vi "保存数据.vi"   [LabVIEW 2016, in "main.lvlib"]
uses:
  main.lvlib
types:
  T1 = typedef "剖面数据_EXO2.ctl" = cluster{"时间":timestamp, "测量模式":string, "数据类型":string, "数据标识":string, "湖面水深":sgl, "缆绳下放长度":sgl, "层数":u16, "row":u16, "水温":sgl, "比电导率":sgl, "电导率":sgl, "盐度":sgl, "总溶解固体":sgl, "pH":sgl, "pHmV":sgl, "ORP":sgl, "饱和度":sgl, "DO":sgl, "浊度":sgl, "叶绿素a":sgl, "蓝绿藻":sgl, "水深":sgl, "设置水深":sgl}
  T2 = typedef "剖面数据_bbe_NAQDO.ctl" = cluster{"时间":timestamp, "测量模式":string, "数据类型":string, "数据标识":string, "湖面水深":sgl, "缆绳下放长度":sgl, "层数":u16, "row":u16, "水温":sgl, "DO":sgl, "饱和度":sgl, "绿藻":sgl, "蓝藻":sgl, "硅甲藻":sgl, "隐藻":sgl, "黄色物质":sgl, "总藻":sgl, "透光率":sgl, "水深":sgl, "设置水深":sgl}
  T3 = cluster{"EXO2 message":T1, "bbe message":T2, "初级生产力":cluster{"时间":timestamp, "设置水深":sgl, "测控模式":u16, "系统状态":u16, "命令集":u16, "测量更新标志":u16, "测量平均次数":u16, "脉冲间歇时间":u16, "PMT增益":u16, "激发诱导光强":u16, "仿真环境光强":u16, "驰豫脉冲脉宽":u16, "驰豫脉冲周期":u16, "暗适应时间":u16, "光适应时间":u16, "系统电压":sgl, "系统温度":sgl, "F0":sgl, "Fm":sgl, "Fv/Fm":sgl, "σPSII":sgl, "τQA":sgl, "F0'":sgl, "Fm'":sgl, "Fv'":sgl, "Fv'/Fm'":sgl, "σPSII’":sgl, "τQA’":sgl, "Chla":sgl, "PAR":sgl, "GPP":sgl, "DF0":sgl, "DFv":sgl}}
  T4 = cluster{"时间":timestamp, "设置水深":sgl, "测控模式":u16, "系统状态":u16, "命令集":u16, "测量更新标志":u16, "测量平均次数":u16, "脉冲间歇时间":u16, "PMT增益":u16, "激发诱导光强":u16, "仿真环境光强":u16, "驰豫脉冲脉宽":u16, "驰豫脉冲周期":u16, "暗适应时间":u16, "光适应时间":u16, "系统电压":sgl, "系统温度":sgl, "F0":sgl, "Fm":sgl, "Fv/Fm":sgl, "σPSII":sgl, "τQA":sgl, "F0'":sgl, "Fm'":sgl, "Fv'":sgl, "Fv'/Fm'":sgl, "σPSII’":sgl, "τQA’":sgl, "Chla":sgl, "PAR":sgl, "GPP":sgl, "DF0":sgl, "DFv":sgl}
  T5 = typedef "checkbox.ctl" = bool
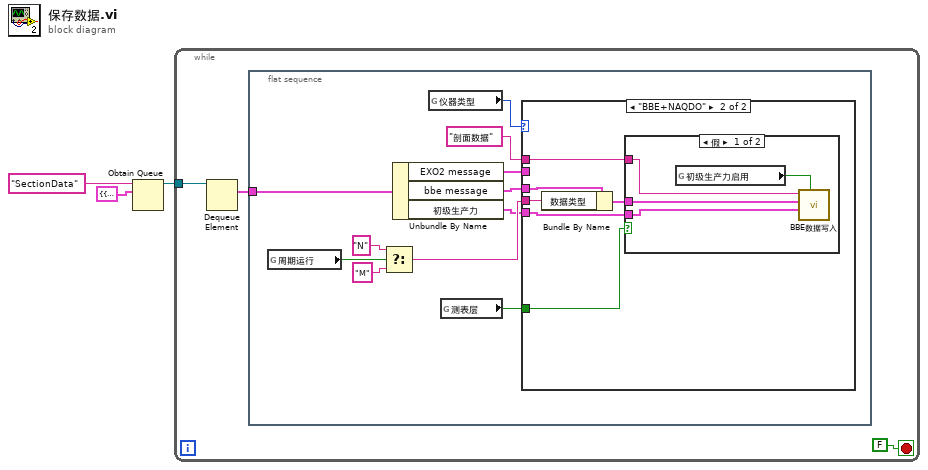
[diagram p0: block diagram]
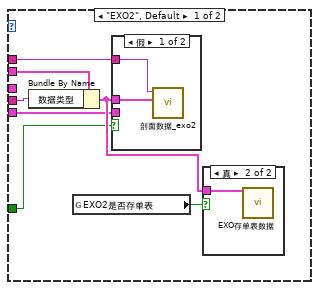
[diagram p2: hidden frame]
diagram:
  n1 = Obtain Queue(name (unnamed)="SectionData" ("名称（未命名）"), element data type=T3 {"EXO2 message"={"时间"=timestamp(0 s since 1904-01-01), "测量模式"="水样测试", "数据类型"="N", "数据标识"="N", "湖面水深"=0.0, "缆绳下放长度"=0.0, "层数"=0, "row"=0, "水温"=0.0, "比电导率"=0.0, "电导率"=0.0, "盐度"=0.0, "总溶解固体"=0.0, "pH"=0.0, "pHmV"=0.0, "ORP"=0.0, "饱和度"=0.0, "DO"=0.0, "浊度"=0.0, "叶绿素a"=0.0, "蓝绿藻"=0.0, "水深"=0.0, "设置水深"=0.0}, "bbe message"={"时间"=timestamp(0 s since 1904-01-01), "测量模式"="水样测试", "数据类型"="N", "数据标识"="N", "湖面水深"=0.0, "缆绳下放长度"=0.0, "层数"=0, "row"=0, "水温"=0.0, "DO"=0.0, "饱和度"=0.0, "绿藻"=0.0, "蓝藻"=0.0, "硅甲藻"=0.0, "隐藻"=0.0, "黄色物质"=0.0, "总藻"=0.0, "透光率"=0.0, "水深"=0.0, "设置水深"=0.0}, "初级生产力"={"时间"=timestamp(0 s since 1904-01-01), "设置水深"=0.0, "测控模式"=0, "系统状态"=0, "命令集"=0, "测量更新标志"=0, "测量平均次数"=0, "脉冲间歇时间"=0, "PMT增益"=0, "激发诱导光强"=0, "仿真环境光强"=0, "驰豫脉冲脉宽"=0, "驰豫脉冲周期"=0, "暗适应时间"=0, "光适应时间"=0, "系统电压"=0.0, "系统温度"=0.0, "F0"=0.0, "Fm"=0.0, "Fv/Fm"=0.0, "σPSII"=0.0, "τQA"=0.0, "F0'"=0.0, "Fm'"=0.0, "Fv'"=0.0, "Fv'/Fm'"=0.0, "σPSII’"=0.0, "τQA’"=0.0, "Chla"=0.0, "PAR"=0.0, "GPP"=0.0, "DF0"=0.0, "DFv"=0.0}} ("簇")) -> (queue out=w2:refnum<queue>)  [unwired: 3 in, 2 out]
  n2 = while {
    tunnel: w2 -> [w6]
    stop <- FALSE stop-if-true
    n3 = Dequeue Element(queue=w6) -> (element=w4:T3)  [unwired: 2 in, 3 out]
    n4 = flat-sequence {
      tunnel: w4 -> [w17]
      frame #0 {
        n5 = global read "全局断电保存变量.vi" "周期运行"() -> (w13:bool)
        n6 = Select(t="N" ("数据类型"), s=w13, f="M" ("数据类型")) -> (s? t:f=w14:string)
        n7 = Unbundle By Name(w17) -> ("EXO2 message"=w10:T1, "bbe message"=w11:T2, "初级生产力"=w7:T4)
        n8 = global read "全局断电保存变量.vi" "仪器类型"() -> (w12:enum16{"EXO2", "BBE+NAQDO", "HL7"})
        n9 = global read "全局非断电保持变量.vi" "测表层"() -> (w8:bool)
        n10 = case shown="\"BBE+NAQDO\"" w12 {
          tunnel: w14 -> [w23 w31]
          tunnel: w11 -> [_ w33]
          tunnel: w10 -> [w24 _]
          tunnel: "剖面数据" ("Tabe Name") -> [w22 w30]
          tunnel: w8 -> [w20 w29]
          tunnel: w7 -> [w18 w28]
          frame "EXO2", Default {
            n11 = Bundle By Name(cluster=w24, "数据类型"=w23) -> (w21:T1)
            n12 = global read "全局断电保存变量.vi" "EXO2是否存单表"() -> (w19:T5)
            n13 = case shown="假" w20 {
              tunnel: w22 -> [w26 _]
              tunnel: w21 -> [w25 _]
              tunnel: w18 -> [_ _]
              frame False {
                n14 = call "剖面数据_exo2.vi"("Tabe Name"=w26, "data"=w25) -> ()  [unwired: 8 in, 1 out]
              }
              frame True {
              }
            }
            n15 = case shown="真" w19 {
              tunnel: w21 -> [_ w27]
              frame False {
              }
              frame True {
                n16 = call "EXO存单表数据.vi"("data"=w27) -> ()  [unwired: 19 in]
              }
            }
          }
          frame "BBE+NAQDO" {
            n17 = Bundle By Name(cluster=w33, "数据类型"=w31) -> (w32:T2)
            n18 = case shown="假" w29 {
              tunnel: w32 -> [w36 _]
              tunnel: w30 -> [w37 _]
              tunnel: w28 -> [w35 _]
              frame False {
                n19 = global read "全局断电保存变量.vi" "初级生产力启用"() -> (w34:T5)
                n20 = call "BBE数据写入.vi"("初级生产力启用"=w34, "初级生产力"=w35, "data"=w36, "Tabe Name"=w37) -> ()  [unwired: 7 in, 1 out]
              }
              frame True {
              }
            }
          }
        }
      }
    }
  }
